vi "Set Source.vi"(0 "TSM Context In":T2, 1 "RFPM Parameters":T1={"Disconnect SG PM Path?"=FALSE, "SG PM Path"=3, "SG Amplitude Settling (dB)"=0.0, "SG Path Optimization Method"=0, "SA PM Path"=3, "SA PM Coupling Path"=3, "SA Amplitude Settling (dB)"=0.0, "SA Path Optimization Method"=0} {"SA Path Optimization Method" items=["Normal", "Optimize for Dynamic Range"]; "SA PM Coupling Path" items=["Auto"=3, "LNA"=2, "Direct"=0, "Coupled"=1]; "SA PM Path" items=["Auto"=3, "Loop"=2, "Gain"=1, "Direct"=0]; "SG Path Optimization Method" items=["Normal", "Optimize for Dynamic Range"]; "SG PM Path" items=["Auto"=3, "Loop"=2, "Gain"=1, "Direct"=0]}, 2 "Enable S2P De-embedding?":bool, 3 "External Offset (dB)":dbl, 5 "Pin":tag, 7 "Frequency (Hz)":dbl, 9 "Power (dBm)":dbl, 11 "error in":errorcluster, 12 "PAPR":dbl, 13 "Runtime Scaling":dbl) -> (4 "TSM Context Out":T2, 6 "External Gain (dB)":dbl, 8 "Digital Gain (dB)":dbl, 10 "Calibrated Power (dBm)":dbl, 14 "RFPM Handle":refnum<k15>, 15 "error out":errorcluster)   [LabVIEW 2023, in "RFFixtureCharact.RFPM.lvlib" / "RF Subsystem Session Provider.lvclass"]
uses:
  RF Subsystem Session Provider.lvclass
  <vilib>/NI_TestStand_SemiconductorModule/NI_TestStand_Semiconductor_Module.lvlibp/PinMap/General/SemiconductorModuleContext.ctl
  Controls/RFPM Parameters.ctl
  <vilib>/NI_TestStand_SemiconductorModule/NI_TestStand_Semiconductor_Module.lvlibp/PinMap/RF/RFPM/PinToNIRFPMSessionsWithPaths.vi
  <instrlib>/niRFPM/niRFPM.llb/NI-RFPM Set TX Path By Switch Path String.vi
  <vilib>/NI_TestStand_SemiconductorModule/NI_TestStand_Semiconductor_Module.lvlibp
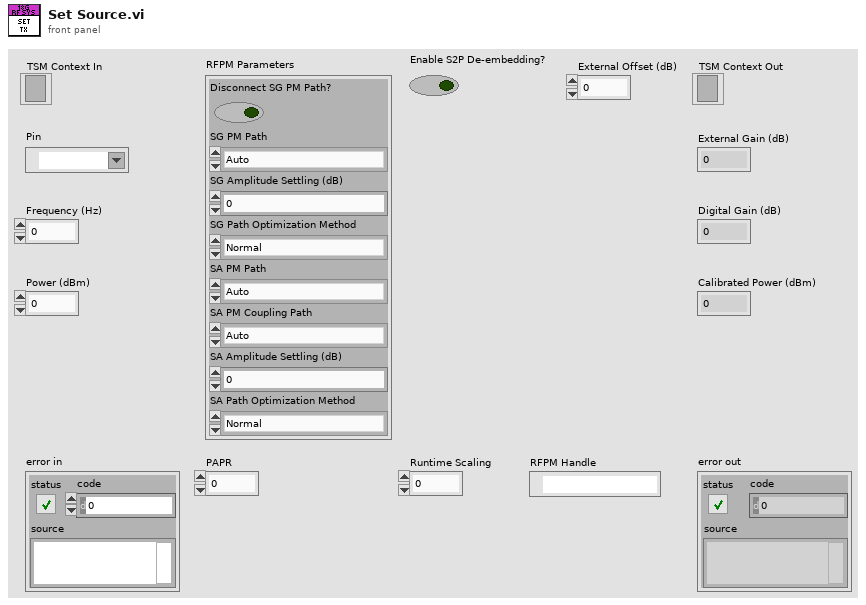
[diagram p1: front panel]
types:
  T1 = typedef "RFFixtureCharact.RFPM.lvlib/RF Subsystem Session Provider.lvclass/RFPM Parameters.ctl" = cluster{"Disconnect SG PM Path?":bool, "SG PM Path":u32, "SG Amplitude Settling (dB)":dbl, "SG Path Optimization Method":i32, "SA PM Path":u32, "SA PM Coupling Path":u32, "SA Amplitude Settling (dB)":dbl, "SA Path Optimization Method":i32}
  T2 = typedef "NI_TestStand_Semiconductor_Module.lvlibp/SemiconductorModuleContext.ctl" = refnum<k7>
  T3 = typedef "NI_TestStand_Semiconductor_Module.lvlibp/DeembeddingFile.ctl" = cluster{" Path":path, "Orientation":i32}
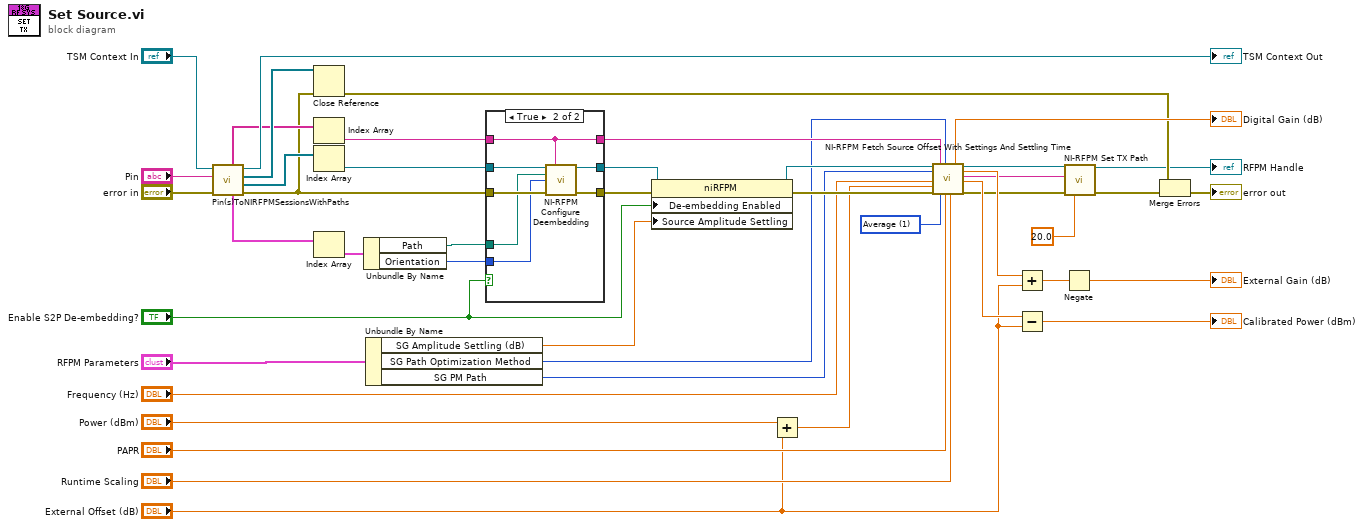
[diagram p0: block diagram]
diagram:
  w27 = 1 items=["Peak", "Average"] ("Power Level Type")
  n1 = call-poly <vilib>:"Pin(s)ToNIRFPMSessionsWithPaths.vi"("error in (no error)"="error in", "Pin"="Pin", "Semiconductor Module Context"="TSM Context In") -> ("error out"=w24:errorcluster, "Instrument Sessions"=w39:refnum<k15>[], "Semiconductor Module Contexts"=w41:T2[], "Semiconductor Module Context out"=→"TSM Context Out":T2, "De-embedding Files"=w38:T3[], "Ports List"=w40:string[])  [unwired: 3 in]
  n2 = Close Reference(reference=w41, error in (no error)=w24) -> (error out=w6:errorcluster)
  n3 = Index Array(array=w40) -> (element=w34:string)  [unwired: 1 in]
  n4 = Index Array(array=w39) -> (element=w36:refnum<k15>)  [unwired: 1 in]
  n5 = Index Array(array=w38) -> (element=w37:T3)  [unwired: 1 in]
  n6 = Unbundle By Name(w37) -> ("Path"=w2:path, "Orientation"=w35:i32)
  n7 = Unbundle By Name("RFPM Parameters") -> ("SG Amplitude Settling (dB)"=w4:dbl, "SG Path Optimization Method"=w5:i32, "SG PM Path"=w29:u32)
  n8 = case shown="True" "Enable S2P De-embedding?" {
    tunnel: w24 -> [w47 w54]
    tunnel: w36 -> [w48 w55]
    tunnel: w35 -> [_ w53]
    tunnel: w34 -> [w46 w50]
    tunnel: [w47 w52] -> w32
    tunnel: [w48 w51] -> w33
    tunnel: [w46 w50] -> w23
    tunnel: w2 -> [_ w49]
    frame False {
    }
    frame True {
      n9 = call <instrlib>:"NI-RFPM Configure Deembedding.vi"("instrument handle"=w55, "port"=w50, "Deembedding S2P File Path"=w49, "Deembedding Orientation"=w53, "error in (no error)"=w54) -> ("instrument handle out"=w51:refnum<k15>, "error out"=w52:errorcluster)  [unwired: 9 in]
    }
  }
  n10 = property class="niRFPM"(reference=w33, error in=w32, "De-embedding Enabled"="Enable S2P De-embedding?", "Source Amplitude Settling"=w4) -> (reference out=w30:refnum<k15>, error out=w31:errorcluster)
  n11 = Add(x="Power (dBm)", y="External Offset (dB)") -> (x+y=w19:dbl)
  n12 = call <instrlib>:"NI-RFPM Fetch Source Offset With Settings And Settling Time.vi"("instrument handle"=w30, "Source Path"=w29, "Frequency"="Frequency (Hz)", "Power"=w19, "error in"=w31, "Port"=w23, "Power Level Type"=w27, "Optimization Method"=w5, "PAPR"="PAPR", "Runtime Scaling"="Runtime Scaling") -> ("Digital Gain"=→"Digital Gain (dB)":dbl, "instrument handle out"=w11:refnum<k15>, "Source Offset"=w18:dbl, "Switch Path String"=w10:string, "Calibrated Power"=w17:dbl, "error out"=w12:errorcluster)  [unwired: 3 in, 1 out]
  n13 = Add(x=w18, y="External Offset (dB)") -> (x+y=w14:dbl)
  n14 = Subtract(x=w17, y="External Offset (dB)") -> (x-y=→"Calibrated Power (dBm)":dbl)
  n15 = Negate(x=w14) -> (-x=→"External Gain (dB)":dbl)
  n16 = call-poly <instrlib>:"NI-RFPM Set TX Path.vi"("instrument handle"=w11, "TX Switch Path"=w10, "error in (no error)"=w12, "timeout"=20.0) -> ("instrument handle out"=→"RFPM Handle":refnum<k15>, "error out"=w8:errorcluster)  [unwired: 10 in]
  n17 = Merge Errors(w6, w8) -> (→"error out":errorcluster)
